vi "DataWrite (SubVI).vi"(9 "Data":dbl, 10 "Address":string, 11 "Select Device":u16) -> (3 "Write frame":string)   [LabVIEW 2020]
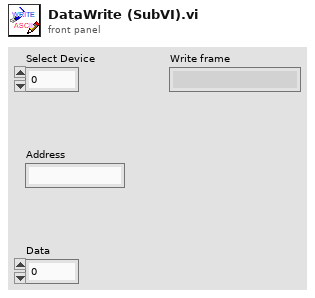
[diagram p1: front panel]
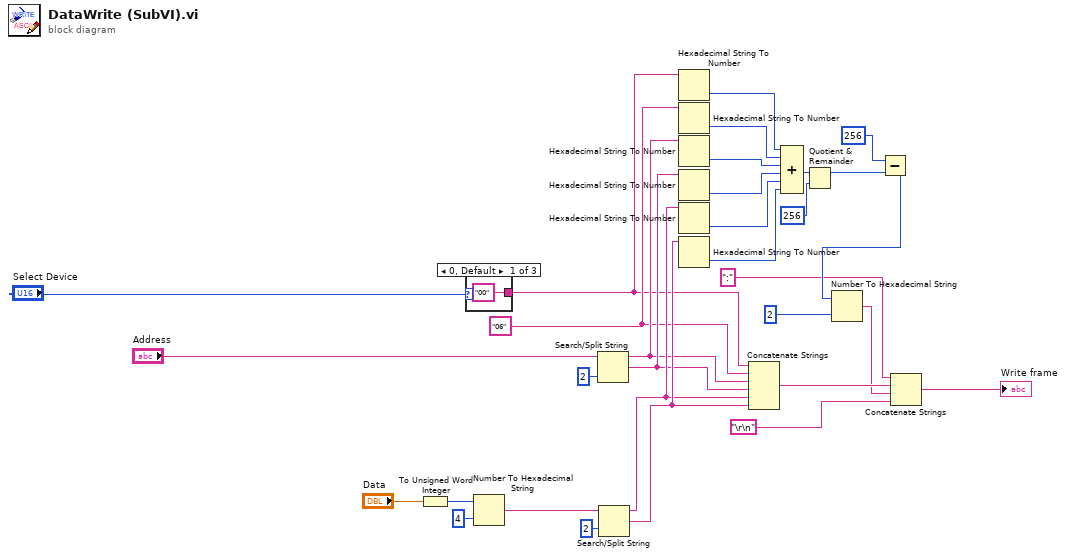
[diagram p0: block diagram]
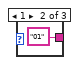
[diagram p2: hidden frame]
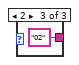
[diagram p3: hidden frame]
diagram:
  w9 = "06" ("string")
  n1 = To Unsigned Word Integer(number="Data") -> (unsigned 16bit integer=w4:u16)
  n2 = case shown="0, Default" "Select Device" {
    tunnel: ["00" ("string") "01" ("string") "02" ("string")] -> w8
    frame 0, Default {
    }
    frame 1 {
    }
    frame 2 {
    }
  }
  n3 = Number To Hexadecimal String(1:i16 4 ("width (-)"), 2:w4) -> (0:w1:string)
  n4 = Search/Split String(string="Address", offset (0)=2) -> (substring before match=w10:string, match + rest of string=w11:string)  [unwired: 1 in, 1 out]
  n5 = Search/Split String(string=w1, offset (0)=2) -> (substring before match=w12:string, match + rest of string=w13:string)  [unwired: 1 in, 1 out]
  n6 = Hexadecimal String To Number(string=w8) -> (number=w14:u32)  [unwired: 2 in, 1 out]
  n7 = Hexadecimal String To Number(string=w9) -> (number=w15:u32)  [unwired: 2 in, 1 out]
  n8 = Hexadecimal String To Number(string=w10) -> (number=w16:u32)  [unwired: 2 in, 1 out]
  n9 = Hexadecimal String To Number(string=w11) -> (number=w17:u32)  [unwired: 2 in, 1 out]
  n10 = Hexadecimal String To Number(string=w12) -> (number=w18:u32)  [unwired: 2 in, 1 out]
  n11 = Hexadecimal String To Number(string=w13) -> (number=w19:u32)  [unwired: 2 in, 1 out]
  n12 = Concatenate Strings(w8, w9, w10, w11, w12, w13) -> (w23:string)
  n13 = Compound Arithmetic op=ADD(w14, w15, w16, w17, w18, w19) -> (w28:u32)
  n14 = Quotient & Remainder(x=w28, y=u32 256) -> (x-y*floor(x/y)=w30:u32)  [unwired: 1 out]
  n15 = Subtract(x=u32 256, y=w30) -> (x-y=w27:u32)
  n16 = Number To Hexadecimal String(1:i16 2 ("width (-)"), 2:w27) -> (0:w21:string)
  n17 = Concatenate Strings(":" ("string"), w23, w21, "\r\n") -> (→"Write frame":string)
